vi "determine_harmonics_NHarmonics.vi"(0 "FFT magnitude":cluster{"f0":dbl, "df":dbl, "magnitude":dbl[]}={"f0"=0.0, "df"=71.42857142857356, "magnitude"=array[7000 elements]}, 1 "FFT phase":cluster{"f0":dbl, "df":dbl, "phase":dbl[]}={"f0"=0.0, "df"=71.42857142857356, "phase"=array[7000 elements]}, 3 "TxRxParams":T1={"sample rate"=1000000.0, "Transmit frequency"=25000.0, "Transmit amplitude"=1.577, "sample rate digital out"=40000.0, "TX cycles"=600, "sample rate DAQ1"=1000000.0, "Receive frequency"=75000.0, "Receive range"=1.0, "TX harmonics"=[50000.0, 75000.0, 100000.0, 125000.0, 150000.0, 175000.0, 200000.0, 225000.0]} {"TX harmonics" format="%#_6p"; "Receive frequency" format="%#_6p"; "sample rate DAQ1" format="%#_6p"; "sample rate digital out" format="%#_6p"; "Transmit frequency" format="%#_6p"; "sample rate" format="%#_6p"}, 4 "TX harmonics mag baseline":dbl[](array[numeric])=[0.0, 0.0, 0.0, 0.0, 0.0, 0.0, 0.0, 0.0, 0.0, 0.0, 0.0, 0.0, 0.0, 0.0, 0.0, 0.0, 0.0, 0.0, 0.0, 0.0, 0.0, 0.0, 0.0, 0.0, 0.0, 0.0, 0.0, 0.0, 0.0, 0.0, 0.0, 0.0, 0.0, 0.0, 0.0, 0.0, 0.0, 0.0, 0.0, 0.0, 0.0, 0.0, 0.0, 0.0, 0.0, 0.0, 0.0, 0.0, 0.0, 0.0, 0.0, 0.0, 0.0, 0.0, 0.0, 0.0, 0.0, 0.0, 0.0, 0.0, 0.0, 0.0, 0.0, 0.0, 0.0, 0.0, 0.0, 0.0, 0.0, 0.0, 0.0, 0.0, 0.0, 0.0, 0.0, 0.0, 0.0, 0.0, 0.0, 0.0, 0.0, 0.0, 0.0, 0.0, 0.0, 0.0, 0.0, 0.0, 0.0, 0.0, 0.0, 0.0, 0.0, 0.0, 0.0, 0.0, 0.0, 0.0, 0.0, 0.0, 0.0], 5 "TX harmonics  phase baseline":dbl[](array[numeric])=[0.0, 0.0, 0.0, 0.0, 0.0, 0.0, 0.0, 0.0, 0.0, 0.0, 0.0, 0.0, 0.0, 0.0, 0.0, 0.0, 0.0, 0.0, 0.0, 0.0, 0.0, 0.0, 0.0, 0.0, 0.0, 0.0, 0.0, 0.0, 0.0, 0.0, 0.0, 0.0, 0.0, 0.0, 0.0, 0.0, 0.0, 0.0, 0.0, 0.0, 0.0, 0.0, 0.0, 0.0, 0.0, 0.0, 0.0, 0.0, 0.0, 0.0, 0.0, 0.0, 0.0, 0.0, 0.0, 0.0, 0.0, 0.0, 0.0, 0.0, 0.0, 0.0, 0.0, 0.0, 0.0, 0.0, 0.0, 0.0, 0.0, 0.0, 0.0, 0.0, 0.0, 0.0, 0.0, 0.0, 0.0, 0.0, 0.0, 0.0, 0.0, 0.0, 0.0, 0.0, 0.0, 0.0, 0.0, 0.0, 0.0, 0.0, 0.0, 0.0, 0.0, 0.0, 0.0, 0.0, 0.0, 0.0, 0.0, 0.0, 0.0], 6 "baseline phase":dbl, 7 "baseline magnitude":dbl) -> (12 "f0 phase":dbl=1.9394134400610221, 13 "f0 mag":dbl=0.024822285377457173, 14 "RX magnitude":dbl=0.0015696795969549263, 15 "RX phase":dbl=0.51499599210196, 18 "mag 2f0-Nf0":dbl[](array[numeric])=[0.07635364629802971, 0.0015696795969549263, 2.5850938198280388e-05, 3.5062095809530066e-05, 2.655041530081199e-05, 3.019279214108981e-05, 1.4173746366290001e-05, 4.367321701979328e-05] format="%#_3p", 19 "phase 2f0-Nf0":dbl[](array[numeric])=[2.093173382122955, 0.51499599210196, -2.573476238721069, 0.1764472036180968, -2.656638672525607, 2.555905242708201, -1.1093217629525705, -0.18697146017335703])   [LabVIEW 2021]
panel:
  out "Rx FFT":cluster{"f0":dbl, "df":dbl, "magnitude":dbl[]}(graph)={"f0"=0.0, "df"=476.1904761905162, "magnitude"=[]}
  out "TX harmonics":dbl[](array[numeric])=[50000.0, 75000.0, 100000.0, 125000.0, 150000.0, 175000.0, 200000.0, 225000.0] format="%#_6p"
  out "RxFreq":dbl=75000.0 format="%#_13g"
  out "TxFreq":dbl=25000.0 format="%#_13g"
  # "Inputs:"
  # "Keep default baseline value under all circumstances zero!!!!"
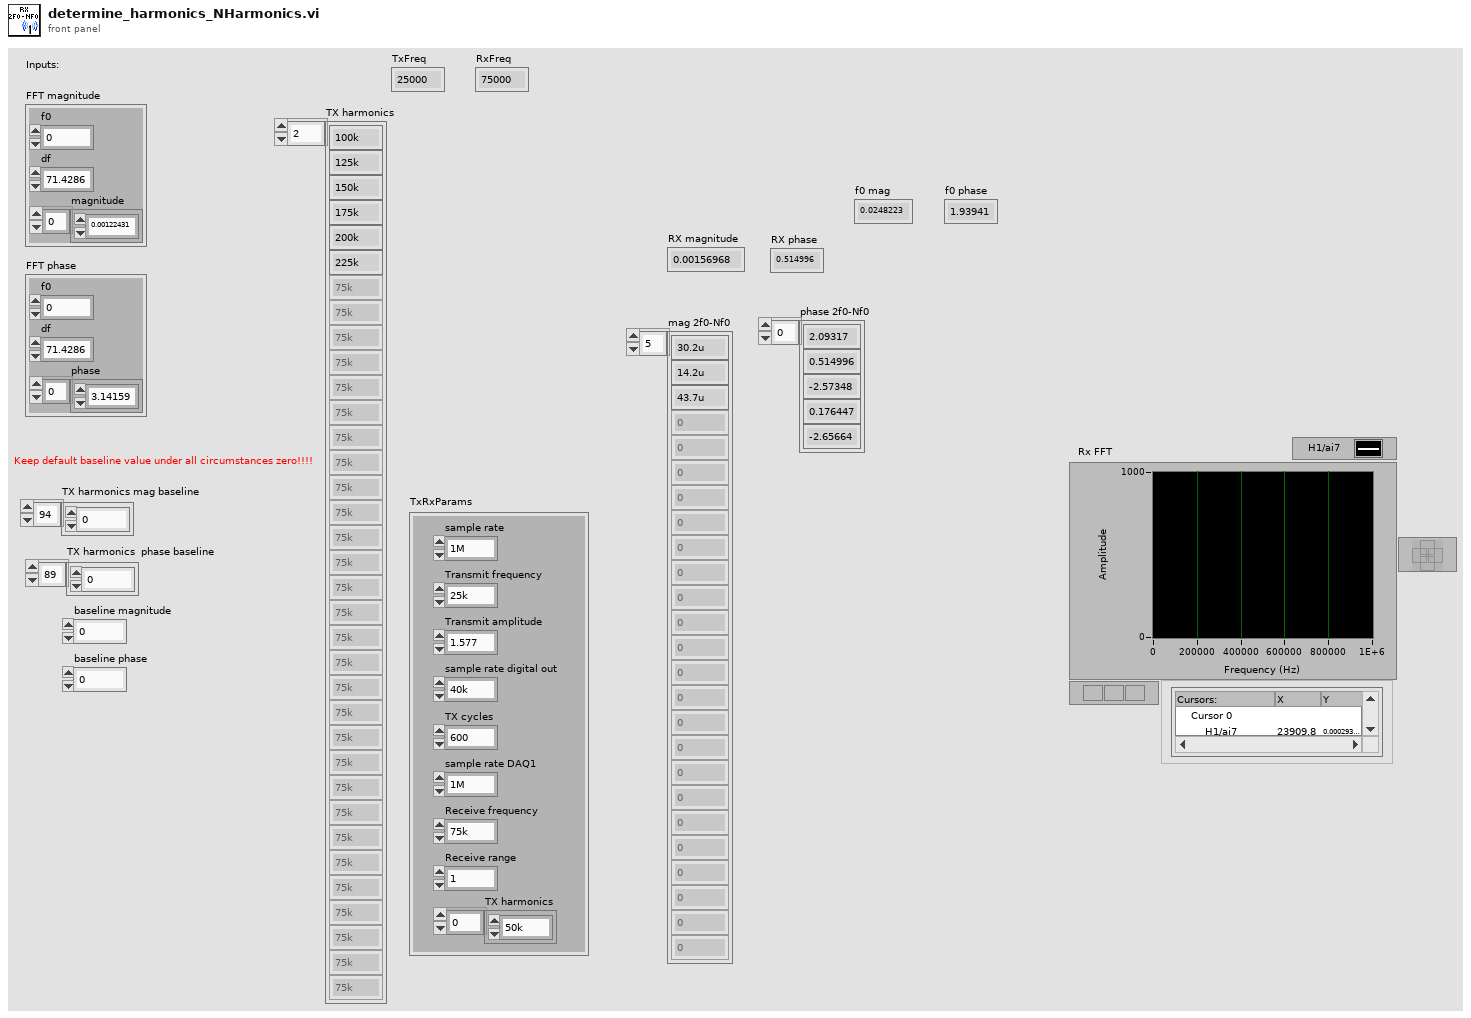
[diagram p1: front panel]
types:
  T1 = cluster{"sample rate":dbl, "Transmit frequency":dbl, "Transmit amplitude":dbl, "sample rate digital out":dbl, "TX cycles":i32, "sample rate DAQ1":dbl, "Receive frequency":dbl, "Receive range":dbl, "TX harmonics":dbl[]}
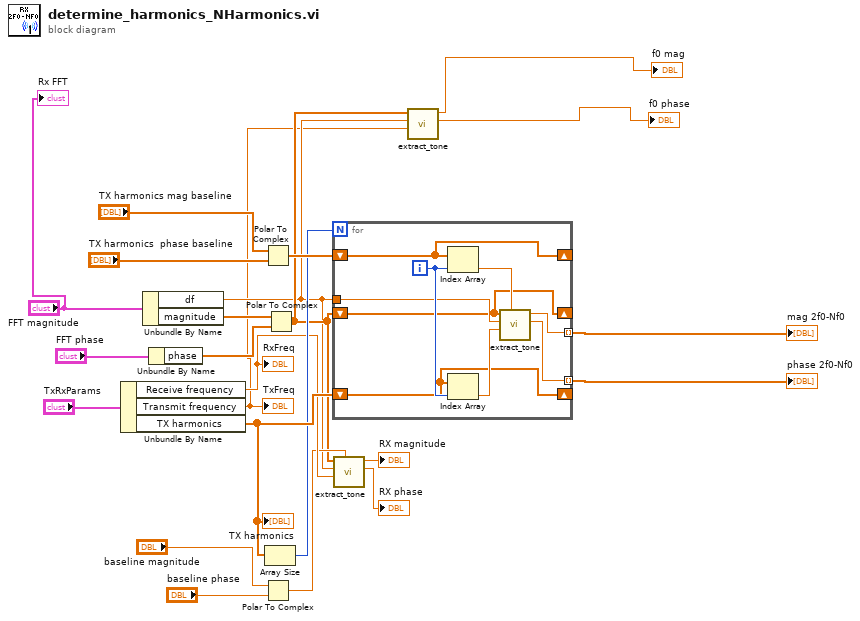
[diagram p0: block diagram]
diagram:
  n1 = Unbundle By Name("TxRxParams") -> ("Receive frequency"=w12:dbl, "Transmit frequency"=w3:dbl, "TX harmonics"=w14:dbl[])
  "TxFreq" <- w3
  "RxFreq" <- w12
  "TX harmonics" <- w14
  n2 = Unbundle By Name("FFT magnitude") -> ("df"=w4:dbl, "magnitude"=w21:dbl[])
  n3 = Unbundle By Name("FFT phase") -> ("phase"=w20:dbl[])
  n4 = Polar To Complex(1:"TX harmonics  phase baseline", 2:"TX harmonics mag baseline") -> (0:w15:cdb[])
  n5 = Polar To Complex(1:"baseline phase", 2:"baseline magnitude") -> (0:w11:cdb)
  n6 = Array Size(array=w14) -> (size(s)=w13:i32)
  n7 = Polar To Complex(1:w20, 2:w21) -> (0:w5:cdb[])
  n8 = for {
    N: w13 -> [_]
    shift-right: [w24] -> _
    shift-left: w15 -> [w24]
    shift-right: [w25] -> _
    shift-left: w14 -> [w25]
    tunnel: [w29] -> w7 mode=indexing
    tunnel: [w28] -> w8 mode=indexing
    tunnel: w4 -> [w27]
    shift-right: [w26] -> _
    shift-left: w5 -> [w26]
    i -> [w32]
    n9 = Index Array(array=w24, index=w32) -> (element=w31:cdb)
    n10 = Index Array(array=w25, index=w32) -> (element=w30:dbl)
    n11 = call "extract_tone.vi"("complex baseline"=w31, "tone frequency [Hz]"=w30, "df"=w27, "complex fft"=w26) -> ("phase (rad)"=w29:dbl, "amplitude"=w28:dbl)  [unwired: 6 in]
  }
  "mag 2f0-Nf0" <- w8
  "phase 2f0-Nf0" <- w7
  n12 = call "extract_tone.vi"("complex baseline"=w11, "tone frequency [Hz]"=w12, "df"=w4, "complex fft"=w5) -> ("phase (rad)"=→"RX phase":dbl, "amplitude"=→"RX magnitude":dbl)  [unwired: 6 in]
  n13 = call "extract_tone.vi"("tone frequency [Hz]"=w3, "df"=w4, "complex fft"=w5) -> ("phase (rad)"=→"f0 phase":dbl, "amplitude"=→"f0 mag":dbl)  [unwired: 7 in]
  "Rx FFT" <- "FFT magnitude"
